vi "read.vi"(8 "error in (no error)":errorcluster, 11 "Lakeshore 331 in":refnum<class "Lakeshore 331.lvclass">) -> (0 "error out":errorcluster, 2 "Data":dbl[](array[numeric]), 3 "Lakeshore 331 out":refnum<class "Lakeshore 331.lvclass">)   [LabVIEW 2022 SP3, in "Lakeshore 331.lvclass"]
uses:
  Lakeshore 331.lvclass
  Lakeshore 331.lvclass/Lakeshore 331.ctl
  Temp Control.lvclass
  <instrlib>/Lake Shore Cryotronics 331/Lake Shore Cryotronics 331.lvlib
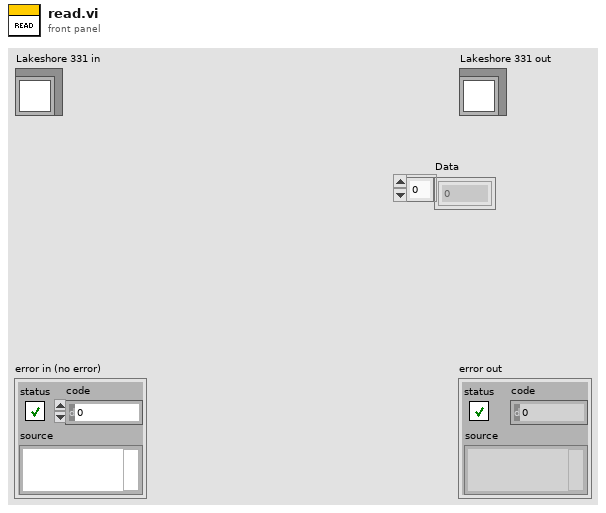
[diagram p1: front panel]
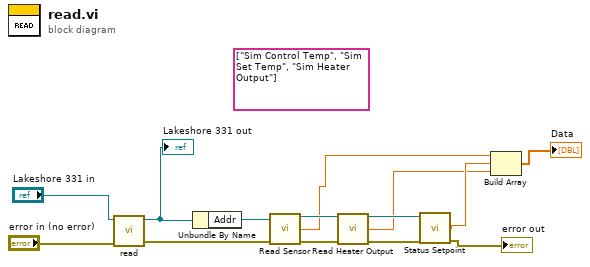
[diagram p0: block diagram]
diagram:
  (unwired) string[] ["Sim Control Temp", "Sim Set Temp", "Sim Heater Output"] ("Channel Names")
  n1 = call-parent "read.vi"("error in (no error)"="error in (no error)", "Temp Control in"="Lakeshore 331 in") -> ("error out"=w2:errorcluster, "Temp Control out"=w12:refnum<class "Lakeshore 331.lvclass">)  [unwired: 7 in, 1 out]
  "Lakeshore 331 out" <- w12
  n2 = Unbundle By Name(w12) -> ("Addr"=w11:refnum<visa-resource-name>)
  n3 = call <instrlib>:"Read Sensor.vi"("VISA resource name"=w11, "error in (no error)"=w2) -> ("VISA resource name out"=w10:refnum<visa-resource-name>, "Kelvin Reading"=w8:dbl, "error out"=w5:errorcluster)  [unwired: 9 in, 2 out]
  n4 = call <instrlib>:"Read Heater Output.vi"("VISA resource name"=w10, "error in (no error)"=w5) -> ("VISA resource name out"=w9:refnum<visa-resource-name>, "Loop 1\nHeater Output"=w6:dbl, "error out"=w4:errorcluster)  [unwired: 11 in]
  n5 = call <instrlib>:"Status Setpoint.vi"("VISA resource name"=w9, "error in (no error)"=w4) -> ("Setpoint"=w7:dbl, "error out"=→"error out":errorcluster)  [unwired: 11 in, 1 out]
  n6 = Build Array(w8, w7, w6) -> (→"Data":dbl[])
